vi "Format table.vi"(11 "Table输入":refnum<vi>) -> ()   [LabVIEW 2016]
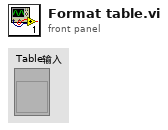
[diagram p1: front panel]
types:
  T1 = cluster{"Font Name:":string, "Size":i16, "Strikeout?":bool, "Italic?":bool, "Underline?":bool, "Outline?":bool, "Shadow?":bool, "Bold?":bool}
  T2 = enum16{"User-specified Font", "Application Font", "System Font", "Dialog Font"}
  T3 = typedef "LVFontTypeDef.ctl" = cluster{"Font Name":string, "Size":u16, "Bold":bool, "Italic":bool, "Underline":bool, "Strikeout":bool, "Color":u32}
  T4 = cluster{"left":i16, "top":i16, "right":i16, "bottom":i16}
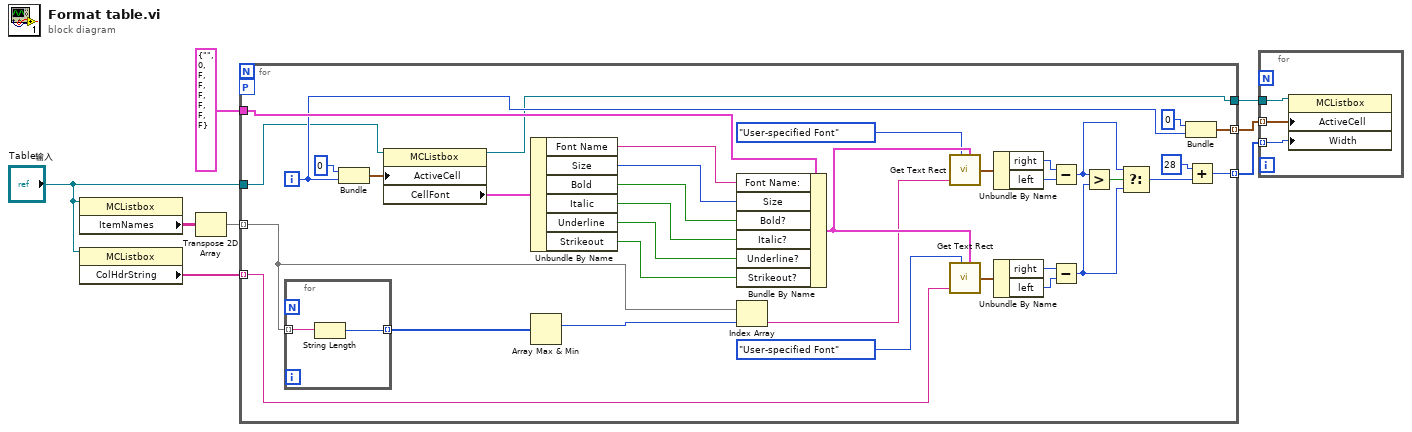
[diagram p0: block diagram]
diagram:
  n1 = property class="MCListbox"(reference="Table输入") -> ("ItemNames"=w8:string[][])  [unwired: 1 in, 2 out]
  n2 = property class="MCListbox"(reference="Table输入") -> ("ColHdrString"=w4:string[])  [unwired: 1 in, 2 out]
  n3 = Transpose 2D Array(2D array=w8) -> (transposed array=w7:string[][])
  n4 = for {
    tunnel: w7 -> [w13] mode=indexing
    tunnel: T1 {"Font Name:"="", "Size"=0, "Strikeout?"=FALSE, "Italic?"=FALSE, "Underline?"=FALSE, "Outline?"=FALSE, "Shadow?"=FALSE, "Bold?"=FALSE} ("[user-specified font]") -> [w43]
    tunnel: "Table输入" -> [w39]
    tunnel: w4 -> [w36] mode=indexing
    workers-P: _ -> [_]
    tunnel: [w29] -> w2 mode=indexing
    tunnel: [w27] -> w1
    tunnel: [w28] -> w3 mode=indexing
    i -> [w42]
    n5 = for {
      tunnel: w13 -> [w45] mode=indexing
      tunnel: [w44] -> w12 mode=indexing
      n6 = String Length(string=w45) -> (length=w44:i32)
    }
    n7 = Bundle(0, w42) -> (w15:cluster{i32, i32})  [unwired: 1 in]
    n8 = property on="属性节点" class="MCListbox"(reference=w39, "ActiveCell"=w15) -> (reference out=w27:refnum<vi>, "CellFont"=w16:T3)  [unwired: 1 in, 1 out]
    n9 = Unbundle By Name(w16) -> ("Font Name"=w26:string, "Size"=w25:u16, "Bold"=w24:bool, "Italic"=w23:bool, "Underline"=w22:bool, "Strikeout"=w21:bool)
    n10 = Array Max & Min(array=w12) -> (max index (indices)=w11:i32)  [unwired: 3 out]
    n11 = Bundle By Name(cluster=w43, "Font Name:"=w26, "Size"=w25, "Bold?"=w24, "Italic?"=w23, "Underline?"=w22, "Strikeout?"=w21) -> (w38:T1)
    n12 = Index Array(array=w13, index=w11) -> (element=w10:string)
    n13 = call <vilib>:"Get Text Rect.vi"("desired font(Application)"=T2."User-specified Font", "text"=w10, "[user-specified font]"=w38) -> ("rect"=w19:T4)  [unwired: 6 in]
    n14 = call <vilib>:"Get Text Rect.vi"("desired font(Application)"=T2."User-specified Font", "text"=w36, "[user-specified font]"=w38) -> ("rect"=w33:T4)  [unwired: 6 in]
    n15 = Unbundle By Name(w19) -> ("right"=w18:i16, "left"=w17:i16)
    n16 = Unbundle By Name(w33) -> ("right"=w34:i16, "left"=w35:i16)
    n17 = Subtract(x=w18, y=w17) -> (x-y=w9:i16)
    n18 = Subtract(x=w34, y=w35) -> (x-y=w31:i16)
    n19 = Greater?(x=w9, y=w31) -> (0:w32:bool)
    n20 = Select(t=w9, s=w32, f=w31) -> (s? t:f=w30:i16)
    n21 = Bundle(0, w42) -> (w28:cluster{i32, i32})  [unwired: 1 in]
    n22 = Add(x=i16 28, y=w30) -> (x+y=w29:i16)
  }
  n23 = for {
    tunnel: w3 -> [w48] mode=indexing
    tunnel: w2 -> [w47] mode=indexing
    tunnel: w1 -> [w46]
    n24 = property on="属性节点" class="MCListbox"(reference=w46, "ActiveCell"=w48, "Width"=w47) -> ()  [unwired: 1 in, 2 out]
  }
